vi "TDMS_strings to file.vi"(4 "property Metadata":variant[](array[variant]), 6 "Channel Names":string[](array[string]), 7 "Group Name":string="A", 8 "error in (no error)":errorcluster, 9 "Data":string[](array[string]), 10 "Measurement":string, 11 "Base path":path) -> (0 "error out":errorcluster, 3 "file out":refnum<k34>)   [LabVIEW 2019]
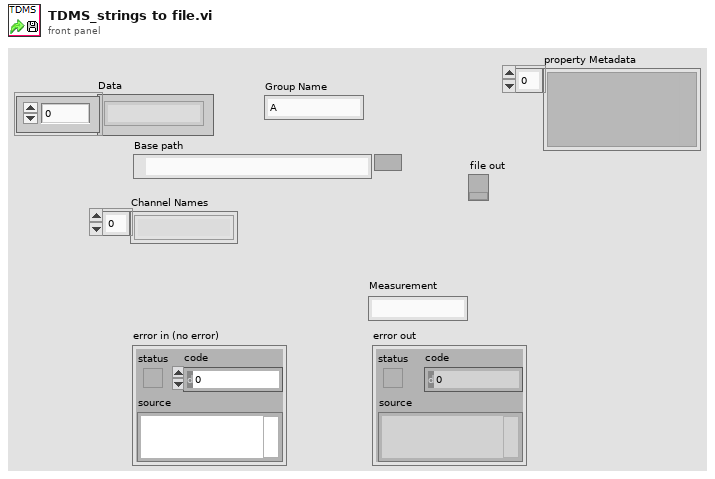
[diagram p1: front panel]
types:
  T1 = enum16{"open", "open or create", "create or replace", "create", "open (read-only)"}
  T2 = typedef "LVDateTimeRec.ctl" = cluster{"fractional second":dbl, "second":i32, "minute":i32, "hour":i32, "day of month":i32, "month":i32, "year":i32, "day of week":i32, "day of year":i32, "DST":i32}
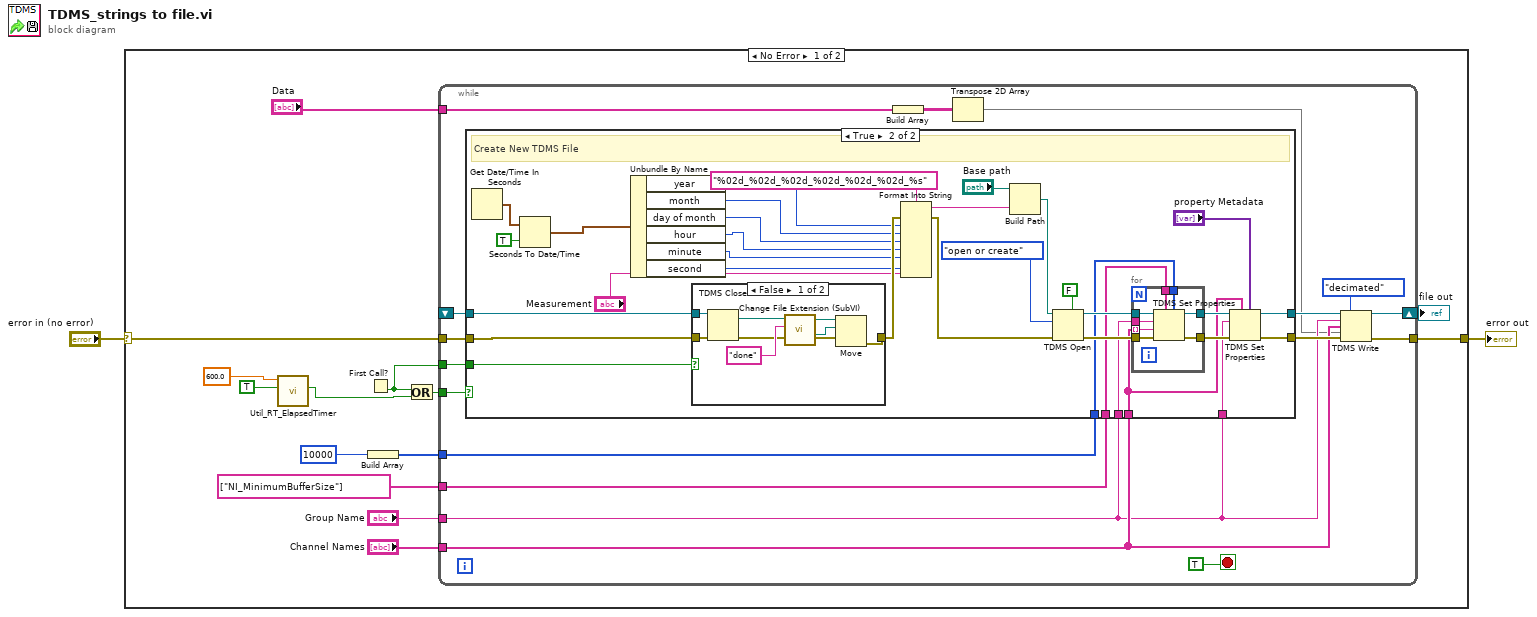
[diagram p0: block diagram]
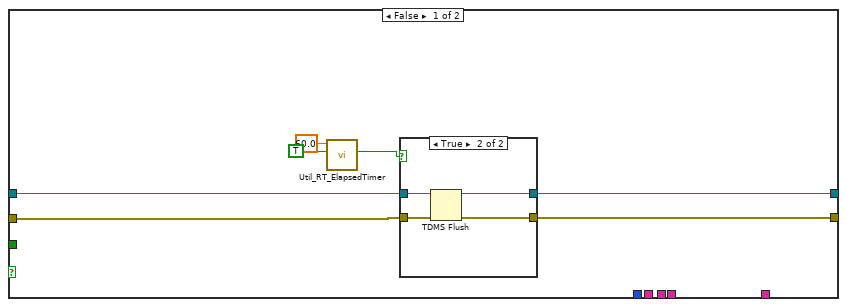
[diagram p2: hidden frame]
diagram:
  n1 = case shown="No Error" "error in (no error)" {
    selector: "error in (no error)" -> [w12 w97]
    tunnel: [w14 w97] -> w2
    frame No Error {
      n2 = call "Util_RT_ElapsedTimer.vi"("Auto Reset"=TRUE, "Target Time (s)"=600.0) -> ("Target\nReached"=w3:bool)  [unwired: 8 in, 1 out]
      n3 = First Call?() -> (First Call?: T/F=w15:bool)
      n4 = Build Array(10000) -> (w9:i32[])
      n5 = Or(x=w15, y=w3) -> (x .or. y?=w16:bool)
      n6 = while {
        tunnel: w16 -> [w33]
        shift-right: [w31] -> w13
        shift-left: _ -> [w32]
        tunnel: w15 -> [w30]
        tunnel: "Data" -> [w25]
        tunnel: [w28] -> w14
        tunnel: w12 -> [w27]
        tunnel: w9 -> [w24]
        tunnel: string[] ["NI_MinimumBufferSize"] ("Channel Names") -> [w23]
        tunnel: "Group Name" -> [w19]
        tunnel: "Channel Names" -> [w20]
        stop <- TRUE stop-if-true
        n7 = case shown="True" w33 {
          tunnel: w32 -> [w40 w74]
          tunnel: w30 -> [_ w75]
          tunnel: [w37 w56] -> w22
          tunnel: w27 -> [w38 w73]
          tunnel: [w39 w57] -> w21
          tunnel: w24 -> [_ w68]
          tunnel: w23 -> [_ w67]
          tunnel: w19 -> [_ w66]
          tunnel: w20 -> [_ w54]
          tunnel: w19 -> [_ w52]
          frame False {
            n8 = call "Util_RT_ElapsedTimer.vi"("Auto Reset"=TRUE, "Target Time (s)"=60.0) -> ("Target\nReached"=w34:bool)  [unwired: 8 in, 1 out]
            n9 = case shown="True" w34 {
              tunnel: w40 -> [w42 w46]
              tunnel: [w42 w45] -> w39
              tunnel: w38 -> [w41 w44]
              tunnel: [w41 w43] -> w37
              frame False {
              }
              frame True {
                n10 = TDMS Flush(4:w44, 7:w46) -> (0:w43:errorcluster, 3:w45:refnum<k34>)
              }
            }
          }
          frame True {
            # "Create New TDMS File"
            n11 = Get Date/Time In Seconds() -> (seconds since 1Jan1904=w50:timestamp)
            n12 = Seconds To Date/Time(time stamp (now)=w50, to UTC (F)=TRUE) -> (date time rec=w48:T2)
            n13 = Unbundle By Name(w48) -> ("year"=w64:i32, "month"=w63:i32, "day of month"=w62:i32, "hour"=w61:i32, "minute"=w60:i32, "second"=w47:i32)
            n14 = case shown="False" w75 {
              tunnel: w74 -> [w95 _]
              tunnel: [w88 w96] -> w79
              tunnel: w73 -> [w94 w96]
              frame False {
                n15 = TDMS Close(8:w94, 11:w95) -> (0:w90:errorcluster, 3:w89:path)
                n16 = call "Change File Extension (SubVI).vi"("New Extension"="done", "appended path"=w89) -> ("New file path"=w91:path, "Original Path"=w93:path)  [unwired: 7 in, 1 out]
                n17 = Move(source path=w93, error in=w90, 10:w91) -> (error out=w88:errorcluster)  [unwired: 2 in, 2 out]
              }
              frame True {
              }
            }
            n18 = Format Into String(format string="%02d_%02d_%02d_%02d_%02d_%02d_%s", error in=w79, w64, w63, w62, w61, w60, w47, "Measurement") -> (resulting string=w65:string, error out=w71:errorcluster)  [unwired: 1 in]
            n19 = Build Path(base path="Base path", name or relative path=w65) -> (appended path=w77:path)
            n20 = TDMS Open(5:FALSE ("create index file? (T)"), 8:w71, 10:T1."open or create" ("operation (0:open)"), 11:w77) -> (0:w70:errorcluster, 3:w69:refnum<k34>)  [unwired: 3 in]
            n21 = for {
              tunnel: w69 -> [w87]
              tunnel: [w86] -> w58
              tunnel: w70 -> [w85]
              tunnel: [w84] -> w55
              tunnel: w67 -> [w83]
              tunnel: w68 -> [w82]
              tunnel: w66 -> [w81]
              tunnel: w54 -> [w80] mode=indexing
              n22 = TDMS Set Properties(5:w82, 7:w83, 8:w85, 9:w80, 10:w81, 11:w87) -> (0:w84:errorcluster, 3:w86:refnum<k34>)  [unwired: 2 out]
            }
            n23 = TDMS Set Properties(5:"property Metadata", 7:w54, 8:w55, 10:w52, 11:w58) -> (0:w56:errorcluster, 3:w57:refnum<k34>)  [unwired: 1 in, 2 out]
          }
        }
        n24 = Build Array(w25) -> (w18:string[][])
        n25 = Transpose 2D Array(2D array=w18) -> (transposed array=w17:string[][])
        n26 = TDMS Write(0:w21, 1:enum16{"decimated", "interleaved"}."decimated" ("data layout (0:decimated)"), 5:w19, 7:w20, 9:w17, 11:w22) -> (4:w31:refnum<k34>, 15:w28:errorcluster)  [unwired: 2 out]
      }
      "file out" <- w13
    }
    frame Error {
    }
  }
  "error out" <- w2
